vi "main.vi"() -> ()   [LabVIEW 2019]
uses:
  <vilib>/silver_ctls/ArrayMatrixCluster/Real Matrix NI_Silver.ctl
  lib/libConvectionDiffusionWrapper/libConvectionDiffusionWrapper.lvlib
panel:
  out "DiffusionValue?":bool
  in  "Stop Button":bool
  in  "Tab Control":enum32{"Control", "Heatmap", "Run Log"}(tab)
  in  "Diffusion Value":dbl=1.0
  in  "Diffusion Switch":enum32{"Value", "Matrix"}(radio)
  in  "Discretization Method":string(combo)="Finite Volumes"
  in  "Source":dbl=1.0
  in  "Reaction Rate":dbl
  in  "Mass Scale":dbl
  in  "Run Button":bool
  in  "Subset":string(combo)="Inner"
  in  "Upwind":string(combo)="Full"
  in  "Grid File":path=path "/home/paul/Schreibtisch/vorlesung-2018/laplace_sample_grid_2d.ugx"
  in  "Solver":string(combo)="Linear Solver"
  in  "Preconditioner":string(combo)="Geometric MultiGrid"
  in  "Max. Iterations":i32=100
  in  "Min. Residuum":dbl=1e-10
  in  "Refinements":i32=3
  in  "Diffusion Matrix Button":bool
  in  "Velocity Vector":dbl[](array[numeric])
  in  "Save As Button":bool
  out "Intensity Graph":dbl[][](graph)
  out "Run Completed":timestamp
  in  "Auto Clear":bool
  in  "Clear Log":bool
  out "Run Log":string
  out "Last Run":timestamp format="%<%x %.3X>T"
  out "Diffusion Matrix":T1
  # "Convection - Diffusion"
  # "Parameter Setup"
  # "Solver Setup"
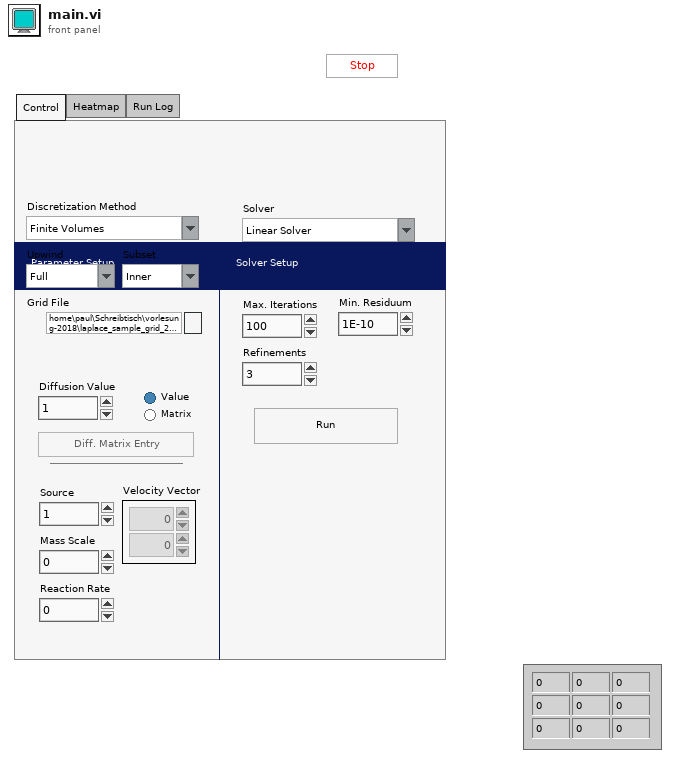
[diagram p1: front panel]
types:
  T1 = typedef "Real Matrix NI_Silver.ctl" = dbl[][]
  T2 = enum8{"Enabled", "Disabled", "Disabled and Grayed Out"}
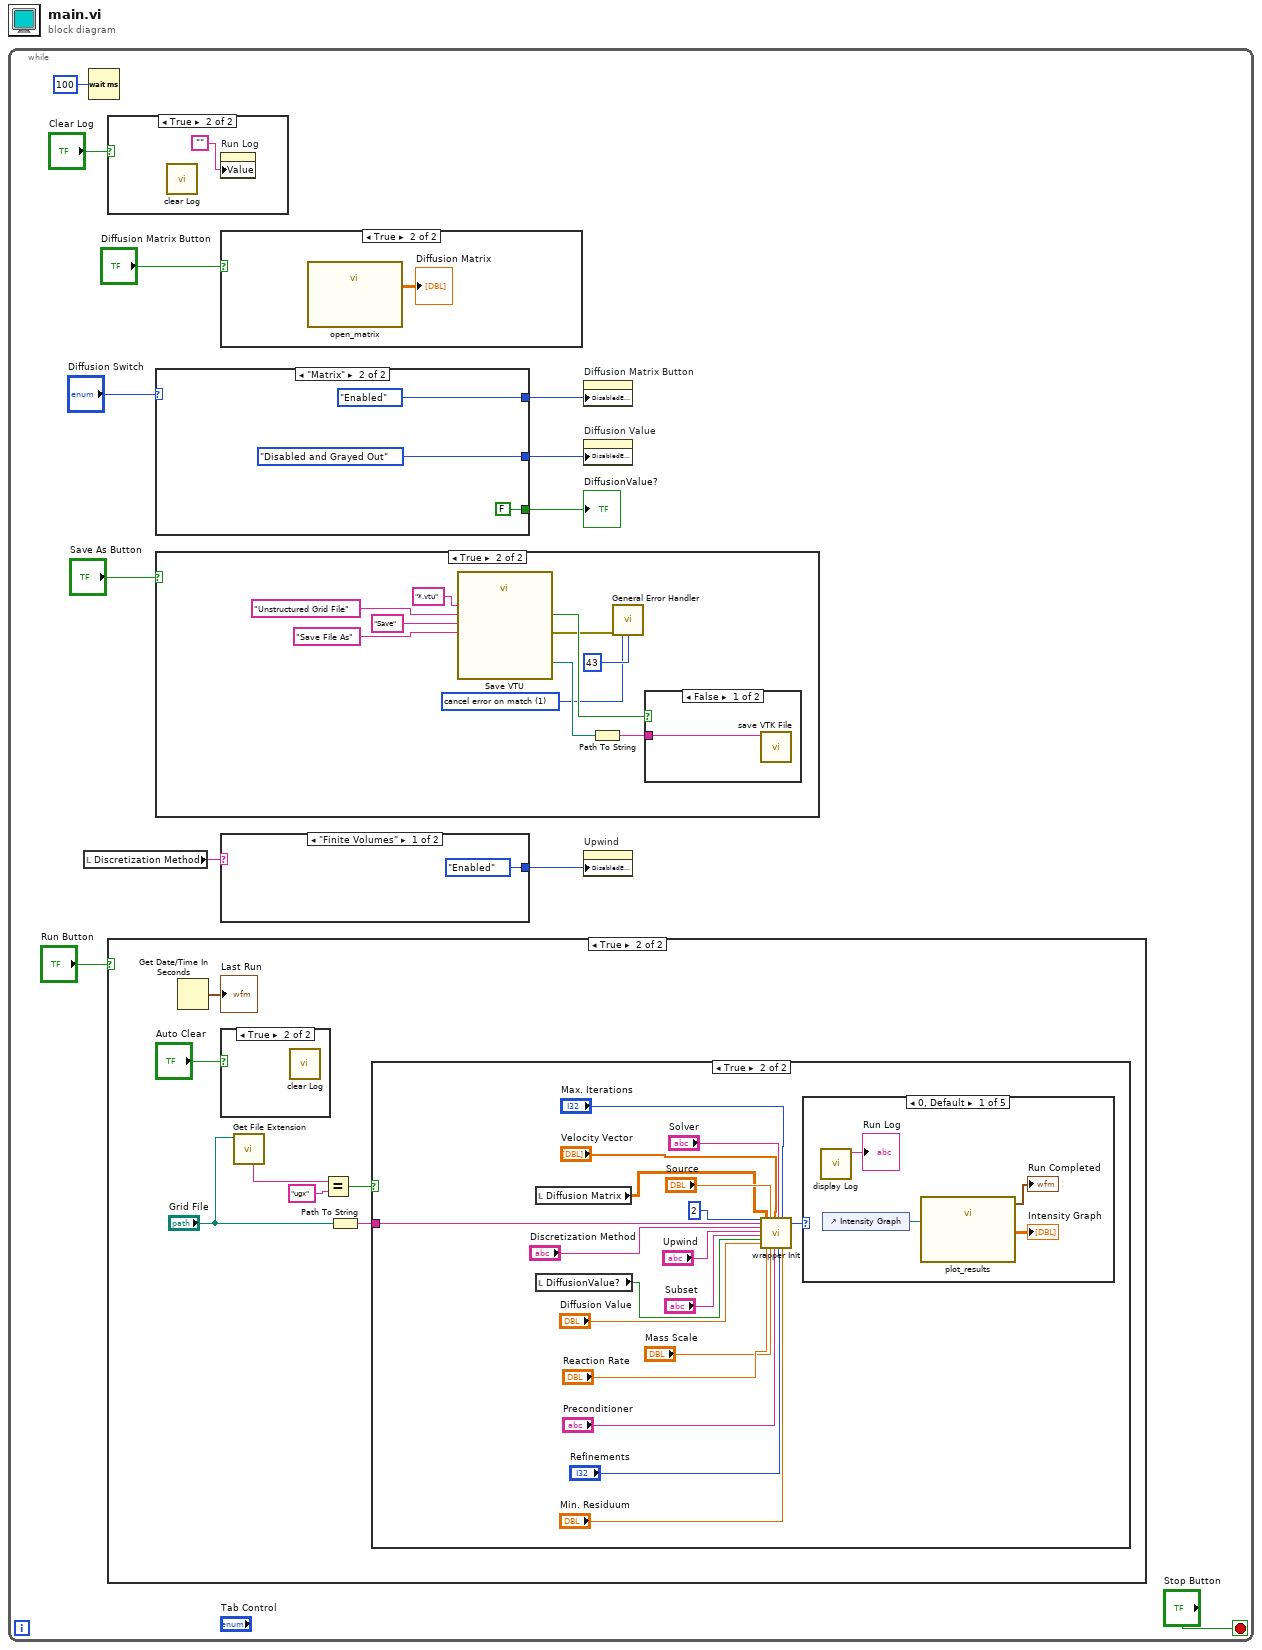
[diagram p0: block diagram]
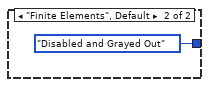
[diagram p6: hidden frame]
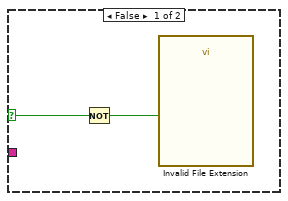
[diagram p9: hidden frame]
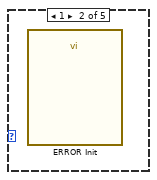
[diagram p10: hidden frame]
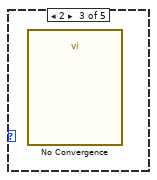
[diagram p11: hidden frame]
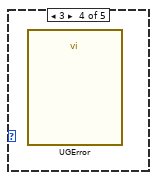
[diagram p12: hidden frame]
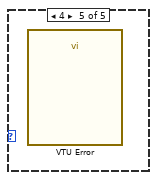
[diagram p13: hidden frame]
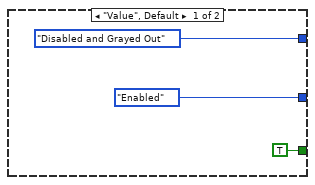
[diagram p14: hidden frame]
diagram:
  n1 = while {
    stop <- "Stop Button" stop-if-true
    n2 = local read "Discretization Method"() -> (w9:string)
    n3 = Wait (ms)(milliseconds to wait=u32 100) -> ()  [unwired: 1 out]
    n4 = case shown="True" "Clear Log" {
      frame False {
      }
      frame True {
        n5 = call "clear Log.vi"() -> ()  [unwired: 11 in, 1 out]
        n6 = property on="Run Log" class="Str"("Value"="") -> ()  [unwired: 2 in, 2 out]
      }
    }
    n7 = case shown="True" "Run Button" {
      frame False {
      }
      frame True {
        n8 = Get Date/Time In Seconds() -> (seconds since 1Jan1904=→"Last Run":timestamp)
        n9 = case shown="True" "Auto Clear" {
          frame False {
          }
          frame True {
            n10 = call "clear Log.vi"() -> ()  [unwired: 11 in, 1 out]
          }
        }
        n11 = call <vilib>:"Get File Extension.vi"("file"="Grid File") -> ("unmodified file extension"=w33:string)  [unwired: 6 in, 4 out]
        n12 = Equal?(x=w33, y="ugx") -> (x = y?=w34:bool)
        n13 = Path To String(path="Grid File") -> (string=w31:string)
        n14 = case shown="True" w34 {
          selector: w34 -> [w35 _]
          tunnel: w31 -> [_ w53]
          frame False {
            n15 = Not(x=w35) -> (.not. x?=w36:bool)
            n16 = call "Invalid File Extension"("Enable"=w36) -> ()  [unwired: 9 in, 2 out]
          }
          frame True {
            n17 = local read "Diffusion Matrix"() -> (w37:T1)
            n18 = local read "DiffusionValue?"() -> (w52:bool)
            n19 = call "wrapper Init.vi"("dim"=2, "fileName"=w53, "discType"="Discretization Method", "upwindType"="Upwind", "subsets"="Subset", "setDiffusionValue"=w52, "diffusionValue"="Diffusion Value", "diffusionMatrix"=w37, "reactionRateValue"="Reaction Rate", "sourceValue"="Source", "massScaleValue"="Mass Scale", "velocityVector"="Velocity Vector", "precondName"="Preconditioner", "solverName"="Solver", "numRefs"="Refinements", "maxNumIter"="Max. Iterations", "absTol"="Min. Residuum") -> ("function return"=w54:i32)  [unwired: 8 in, 2 out]
            n20 = case shown="0, Default" w54 {
              frame 0, Default {
                n21 = call "display Log.vi"() -> ("function return"=→"Run Log":string)  [unwired: 10 in, 1 out]
                n22 = control-ref of="Intensity Graph"() -> (w58:refnum<vi>)
                n23 = call "plot_results.vi"("IntensityGraph in"=w58) -> ("Intensity Graph"=→"Intensity Graph":dbl[][], "Run Completed"=→"Run Completed":timestamp)  [unwired: 9 in]
              }
              frame 1 {
                n24 = call "ERROR Init"() -> ()  [unwired: 10 in, 2 out]
              }
              frame 2 {
                n25 = call "No Convergence"() -> ()  [unwired: 10 in, 2 out]
              }
              frame 3 {
                n26 = call "UGError"() -> ()  [unwired: 10 in, 2 out]
              }
              frame 4 {
                n27 = call "VTU Error"() -> ()  [unwired: 10 in, 2 out]
              }
            }
          }
        }
      }
    }
    n28 = case shown="\"Matrix\"" "Diffusion Switch" {
      tunnel: [T2."Enabled" ("Disabled") T2."Disabled and Grayed Out" ("Disabled")] -> w12
      tunnel: [T2."Disabled and Grayed Out" ("Disabled") T2."Enabled" ("Disabled")] -> w7
      tunnel: [TRUE FALSE] -> w1
      frame "Value", Default {
      }
      frame "Matrix" {
      }
    }
    "DiffusionValue?" <- w1
    n29 = case shown="True" "Save As Button" {
      frame False {
      }
      frame True {
        w13 = 1 items=["no exception", "cancel error on match", "set error on match"] ("[exception action] (none:0)")
        n30 = call "Save VTU"("prompt"="Save File As", "button label"="Save", "pattern (all files)"="*.vtu", "pattern label"="Unstructured Grid File") -> ("selected path"=w17:path, "cancelled"=w18:bool, "error out"=w15:errorcluster)  [unwired: 8 in, 1 out]
        n31 = Path To String(path=w17) -> (string=w16:string)
        n32 = call <vilib>:"General Error Handler.vi"("error in (no error)"=w15, "[exception action] (none:0)"=w13, "[exception code]"=43) -> ()  [unwired: 8 in, 5 out]
        n33 = case shown="False" w18 {
          tunnel: w16 -> [w23 _]
          frame False {
            n34 = call "save VTK File.vi"("path"=w23) -> ()  [unwired: 10 in, 1 out]
          }
          frame True {
          }
        }
      }
    }
    n35 = case shown="True" "Diffusion Matrix Button" {
      frame False {
      }
      frame True {
        n36 = call "open_matrix.vi"() -> ("Output Matrix"=→"Diffusion Matrix":T1)  [unwired: 7 in]
      }
    }
    n37 = case shown="\"Finite Volumes\"" w9 {
      tunnel: [T2."Enabled" ("Disabled") T2."Disabled and Grayed Out" ("Disabled")] -> w8
      frame "Finite Volumes" {
      }
      frame "Finite Elements", Default {
      }
    }
    n38 = property on="Diffusion Matrix Button" class="Bool"("DisabledEnum"=w7) -> ()  [unwired: 2 in, 2 out]
    n39 = property on="Diffusion Value" class="DigNum (strict)"("DisabledEnum"=w12) -> ()  [unwired: 2 in, 2 out]
    n40 = property on="Upwind" class="CmbBox"("DisabledEnum"=w8) -> ()  [unwired: 2 in, 2 out]
  }
